vi "ELVIS III v1.0 Shutdown DIO.vi"(8 "error in (no error)":errorcluster, 10 "Channel List":T3, 11 "myRIO Ref In":T1) -> (0 "error out":errorcluster, 3 "myRIO Ref Out":T1)   [LabVIEW 2021]
uses:
  <vilib>/myRIO/Common/Instrument Driver Framework/myRIO v1.0/DIO/typedefs/DIO Channels List.ctl
  <vilib>/myRIO/Common/Instrument Driver Framework/myRIO v1.0/DIO/typedefs/DIO Channels Enum.ctl
  <vilib>/myRIO/Common/Instrument Driver Framework/Utilities/typedefs/myRIO v1.0 Reference.ctl
  <vilib>/myRIO/Common/Instrument Driver Framework/Utilities/typedefs/Generic FPGA Reference.ctl
  <vilib>/myRIO/Common/Instrument Driver Framework/ELVIS III v1.0/DIO/typedefs/ELVIS III DIO FPGA Reference.ctl
  <vilib>/myRIO/Common/Instrument Driver Framework/ELVIS III v1.0/DIO/typedefs/ELVIS III DIO Bank Enum.ctl
  <vilib>/Utility/error.llb/Error Cluster From Error Code.vi
  <vilib>/rvi/errors/niLvFpgaAdjustHostInterfaceError.vi
  <vilib>/rvi/interface/nirviReadWriteControl/nirviReadWriteControl.xnode
  NiFpgaLv.dll
  <vilib>/rvi/interface/Simulation/niFpgaSimulationCallBeginRW.vi
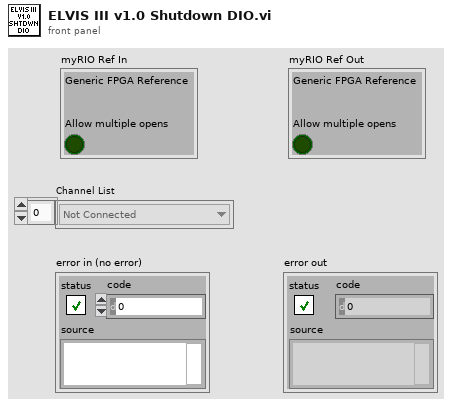
[diagram p1: front panel]
types:
  T1 = typedef "myRIO v1.0 Reference.ctl" = cluster{"Generic FPGA Reference":T2, "Allow multiple opens":bool}
  T2 = typedef "Generic FPGA Reference.ctl" = refnum<k20>
  T3 = typedef "DIO Channels List.ctl" = T4[]
  T4 = typedef "DIO Channels Enum.ctl" = enum16{"Not Connected", "C/DIO0", "C/DIO1", "C/DIO2", "C/DIO3", "C/DIO4", "C/DIO5", "C/DIO6", "C/DIO7", "A/DIO0", "A/DIO1", "A/DIO2", "A/DIO3", "A/DIO4", "A/DIO5", "A/DIO6", "A/DIO7", "A/DIO8", "A/DIO9", "A/DIO10", "A/DIO11", "A/DIO12", "A/DIO13", "A/DIO14", "A/DIO15", "A/DIO16", "A/DIO17", "A/DIO18", "A/DIO19", "B/DIO0", "B/DIO1", "B/DIO2", "B/DIO3", "B/DIO4", "B/DIO5", "B/DIO6", "B/DIO7", "B/DIO8", "B/DIO9", "B/DIO10", "B/DIO11", "B/DIO12", "B/DIO13", "B/DIO14", "B/DIO15", "B/DIO16", "B/DIO17", "B/DIO18", "B/DIO19", "LED0", "LED1", "LED2", "LED3", "Button0", "DIO/DIO0", "DIO/DIO1", "DIO/DIO2", "DIO/DIO3", "DIO/DIO4", "DIO/DIO5", "DIO/DIO6", "DIO/DIO7", "DIO/DIO8", "DIO/DIO9", "SPI/CS0", "SPI/CS1", "SPI/CS2", "SPI/CS3", "LED RADIO (Green)", "LED RADIO (Red)", "LED COMM (Green)", "LED COMM (Red)", "LED MODE (Green)", "LED MODE (Red)"}
  T5 = typedef "ELVIS III DIO Bank Enum.ctl" = enum32{"None", "A/DIO19:0", "B/DIO19:0", "LED3:0", "Button0"}
  T6 = typedef "ELVIS III DIO FPGA Reference.ctl" = refnum<k20>
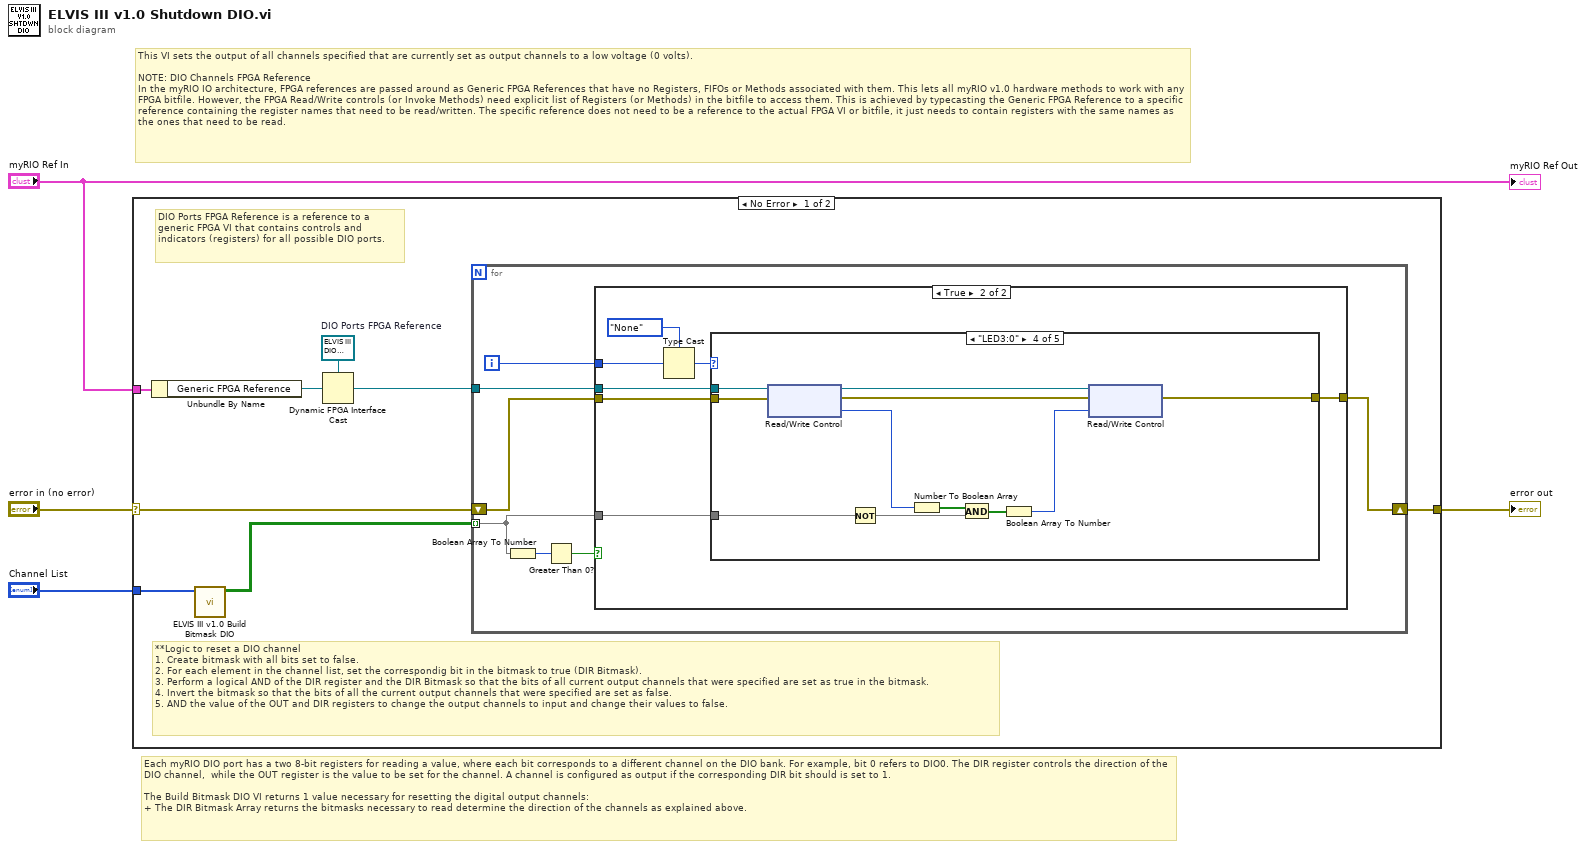
[diagram p0: block diagram]
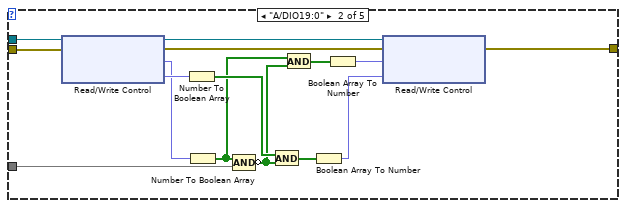
[diagram p4: hidden frame]
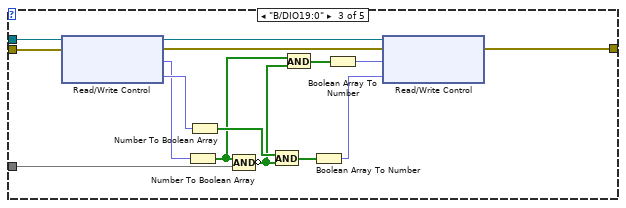
[diagram p5: hidden frame]
diagram:
  # "Each myRIO DIO port has a two 8-bit registers for reading a value, where each bit corresponds to a different channel on the DIO bank. For example, bit 0 refers to DIO0. The DIR register controls the direction of the DIO channel,  while the OUT register is the value to be set for the channel. A channel is configured as output if the corresponding DIR bit should is set to 1.\n\nThe Build Bitmask DIO VI returns 1 value necessary for resetting the digital output channels:\n+ The DIR Bitmask Array returns the bitmasks necessary to read determine the direction of the channels as explained above."
  # "This VI sets the output of all channels specified that are currently set as output channels to a low voltage (0 volts).\n\nNOTE: DIO Channels FPGA Reference\nIn the myRIO IO architecture, FPGA references are passed around as Generic FPGA References that have no Registers, FIFOs or Methods associated with them. This lets all myRIO v1.0 hardware methods to work with any FPGA bitfile. However, the FPGA Read/Write controls (or Invoke Methods) need explicit list of Registers (or Methods) in the bitfile to access them. This is achieved by typecasting the Generic FPGA Reference to a specific reference containing the register names that need to be read/written. The specific reference does not need to be a reference to the actual FPGA VI or bitfile, it just needs to contain registers with the same names as the ones that need to be read."
  n1 = case shown="No Error" "error in (no error)" {
    selector: "error in (no error)" -> [w7 w70]
    tunnel: "myRIO Ref In" -> [w6 _]
    tunnel: [w10 w70] -> w3
    tunnel: "Channel List" -> [w9 _]
    frame No Error {
      w12 = T6 refnum  # DIO Ports FPGA Reference
      # "**Logic to reset a DIO channel\n1. Create bitmask with all bits set to false.\n2. For each element in the channel list, set the correspondig bit in the bitmask to true (DIR Bitmask).\n3. Perform a logical AND of the DIR register and the DIR Bitmask so that the bits of all current output channels that were specified are set as true in the bitmask.\n4. Invert the bitmask so that the bits of all the current output channels that were specified are set as false.\n5. AND the value of the OUT and DIR registers to change the output channels to input and change their values to false."
      # "DIO Ports FPGA Reference is a reference to a generic FPGA VI that contains controls and indicators (registers) for all possible DIO ports."
      n2 = Unbundle By Name(w6) -> ("Generic FPGA Reference"=w5:T2)
      n3 = call <vilib>:"ELVIS III v1.0 Build Bitmask DIO.vi"("Channel List"=w9) -> ("DIR Bitmask Array"=w8:bool[][])  [unwired: 8 in, 2 out]
      n4 = Dynamic FPGA Interface Cast(Session In=w12, Type=w5) -> (Session Out=w11:T6)
      n5 = for {
        tunnel: w8 -> [w13] mode=indexing
        tunnel: w11 -> [w19]
        shift-right: [w17] -> w10
        shift-left: w7 -> [w16]
        i -> [w18]
        n6 = Boolean Array To Number(Boolean array=w13) -> (number=w14:u8)
        n7 = Greater Than 0?(x=w14) -> (x > 0?=w15:bool)
        n8 = case shown="True" w15 {
          tunnel: w19 -> [_ w27]
          tunnel: w18 -> [_ w26]
          tunnel: w13 -> [_ w23]
          tunnel: [w20 w22] -> w17
          tunnel: w16 -> [w20 w21]
          frame False {
          }
          frame True {
            n9 = Type Cast(type=ELVIS_III_DIO_Bank_Enum."None" ("DIO Bank Enum"), x=w26) -> (*(type *) &x=w24:T5)
            n10 = case shown="\"LED3:0\"" w24 {
              tunnel: w27 -> [_ w43 w58 w63 _]
              tunnel: w23 -> [_ w39 w54 w60 _]
              tunnel: [w28 w29 w44 w61 _] -> w22
              tunnel: w21 -> [w28 w42 w57 w62 _]
              frame "None", Default {
              }
              frame "A/DIO19:0" {
                n11 = xnode "Read/Write Control"("FPGA VI Reference In"=w43, "error in"=w42) -> ("FPGA VI Reference Out"=w41:T6, "error out"=w40:errorcluster, "DIO.A_19:0.DIR"=w34:fxp<+,20,20>, "DIO.A_19:0.OUT"=w38:fxp<+,20,20>)
                n12 = Number To Boolean Array(number=w38) -> (Boolean array=w37:bool[])
                n13 = Number To Boolean Array(number=w34) -> (Boolean array=w33:bool[])
                n14 = Compound Arithmetic op=AND(w33, w39) -> (invert w32:bool[])
                n15 = And(x=w37, y=w32) -> (x .and. y?=w36:bool[])
                n16 = And(x=w33, y=w32) -> (x .and. y?=w31:bool[])
                n17 = Boolean Array To Number(Boolean array=w36) -> (number=w35:fxp<+,20,20>)
                n18 = Boolean Array To Number(Boolean array=w31) -> (number=w30:fxp<+,20,20>)
                n19 = xnode "Read/Write Control"("FPGA VI Reference In"=w41, "error in"=w40, "DIO.A_19:0.DIR"=w30, "DIO.A_19:0.OUT"=w35) -> ("error out"=w29:errorcluster)  [unwired: 1 out]
              }
              frame "B/DIO19:0" {
                n20 = xnode "Read/Write Control"("FPGA VI Reference In"=w58, "error in"=w57) -> ("FPGA VI Reference Out"=w56:T6, "error out"=w55:errorcluster, "DIO.B_19:0.DIR"=w49:fxp<+,20,20>, "DIO.B_19:0.OUT"=w53:fxp<+,20,20>)
                n21 = Number To Boolean Array(number=w49) -> (Boolean array=w48:bool[])
                n22 = Number To Boolean Array(number=w53) -> (Boolean array=w52:bool[])
                n23 = Compound Arithmetic op=AND(w48, w54) -> (invert w47:bool[])
                n24 = And(x=w52, y=w47) -> (x .and. y?=w51:bool[])
                n25 = And(x=w48, y=w47) -> (x .and. y?=w46:bool[])
                n26 = Boolean Array To Number(Boolean array=w51) -> (number=w50:fxp<+,20,20>)
                n27 = Boolean Array To Number(Boolean array=w46) -> (number=w45:fxp<+,20,20>)
                n28 = xnode "Read/Write Control"("FPGA VI Reference In"=w56, "error in"=w55, "DIO.B_19:0.DIR"=w45, "DIO.B_19:0.OUT"=w50) -> ("error out"=w44:errorcluster)  [unwired: 1 out]
              }
              frame "LED3:0" {
                n29 = xnode "Read/Write Control"("FPGA VI Reference In"=w63, "error in"=w62) -> ("FPGA VI Reference Out"=w69:T6, "error out"=w68:errorcluster, "DO.LED3:0"=w67:u8)
                n30 = Not(x=w60) -> (.not. x?=w59:bool[])
                n31 = Number To Boolean Array(number=w67) -> (Boolean array=w66:bool[])
                n32 = And(x=w66, y=w59) -> (x .and. y?=w65:bool[])
                n33 = Boolean Array To Number(Boolean array=w65) -> (number=w64:u8)
                n34 = xnode "Read/Write Control"("FPGA VI Reference In"=w69, "error in"=w68, "DO.LED3:0"=w64) -> ("error out"=w61:errorcluster)  [unwired: 1 out]
              }
              frame "Button0" {
              }
            }
          }
        }
      }
    }
    frame Error {
    }
  }
  "error out" <- w3
  "myRIO Ref Out" <- "myRIO Ref In"
